vi "Indexer Closed Loop Control.vi"(10 "Indexer backward":bool, 11 "Indexer Forward":bool) -> (3 "Output PWM":dbl)   [LabVIEW 2011]
uses:
  <vilib>/addons/control/pid/NI_PID_pid.lvlib
  <vilib>/addons/control/pid/pid.llb/PID (DBL).vi
panel:
  out "RPM Error Sampled":dbl
  out "Encoder Sample Spped":dbl
  in  "D":dbl
  in  "I":dbl
  in  "P":dbl
  out "RPM Error":dbl
  out "Encoder Set Speed":dbl
  out "Actual Encoder Speed":dbl
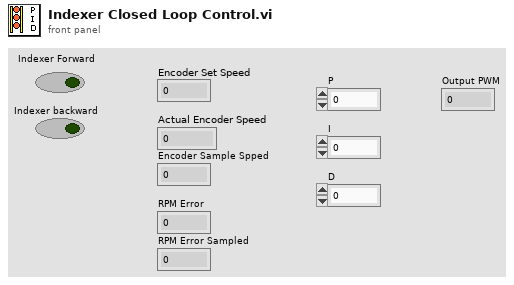
[diagram p1: front panel]
types:
  T1 = typedef "WPI_EncoderDevRef.ctl" = cluster{"DevStatus":errorcluster, "EncoderIndex":T2, "CounterIndex":T3, "DistancePerCount":dbl, "Decoding Type":T4}
  T2 = typedef "FPGA_EncoderIdx.ctl" = enum8{"Enc 0", "Enc 1", "Enc 2", "Enc 3", "Invalid"}
  T3 = typedef "FPGA_CounterCtrSystemIndex.ctl" = enum8{"Ctr 0", "Ctr 1", "Ctr 2", "Ctr 3", "Ctr 4", "Ctr 5", "Ctr 6", "Ctr 7", "Invalid"}
  T4 = typedef "WPI_EncoderType.ctl" = enum16{"1x", "2x", "4x"}
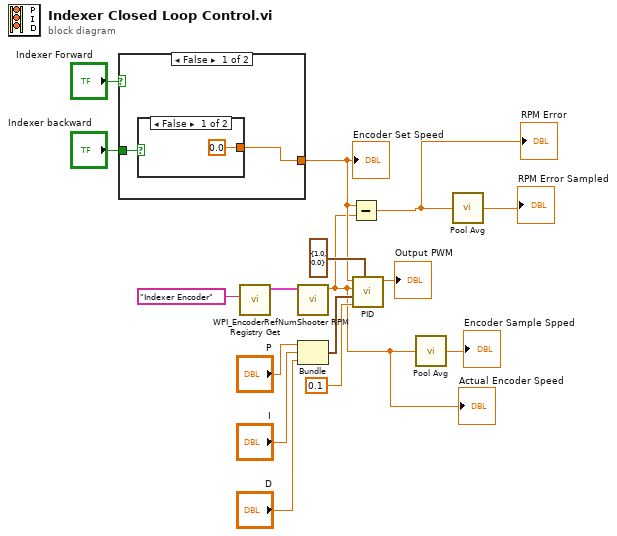
[diagram p0: block diagram]
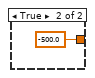
[diagram p2: hidden frame]
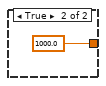
[diagram p3: hidden frame]
diagram:
  n1 = case shown="False" "Indexer Forward" {
    tunnel: [w17 1000.0] -> w11
    tunnel: "Indexer backward" -> [w18 _]
    frame False {
      n2 = case shown="False" w18 {
        tunnel: [0.0 -500.0] -> w17
        frame False {
        }
        frame True {
        }
      }
    }
    frame True {
    }
  }
  "Encoder Set Speed" <- w11
  n3 = call <vilib>:"WPI_EncoderRefNum Registry Get.vi"("refnum name"="Indexer Encoder") -> ("EncoderDevRef"=w6:T1)  [unwired: 9 in, 1 out]
  n4 = call "Shooter RPM.vi"(11:w6) -> ("RPM Output"=w1:dbl)  [unwired: 10 in]
  "Actual Encoder Speed" <- w1
  n5 = Bundle("P"="P", "I"="I", "D"="D") -> (w10:cluster{"P":dbl, "I":dbl, "D":dbl})  [unwired: 1 in]
  n6 = Subtract(x=w11, y=w1) -> (x-y=w3:dbl)
  "RPM Error" <- w3
  n7 = call-poly <vilib>:"PID.vi"("output range"=cluster{"output high":dbl, "output low":dbl} {"output high"=1.0, "output low"=0.0}, "dt (s)"=0.1, "PID gains"=w10, "process variable"=w1, "setpoint"=w11) -> ("output"=→"Output PWM":dbl)  [unwired: 5 in, 1 out]
  n8 = call "Pool Avg.vi"("Input"=w1) -> ("Output Avg"=→"Encoder Sample Spped":dbl)
  n9 = call "Pool Avg.vi"("Input"=w3) -> ("Output Avg"=→"RPM Error Sampled":dbl)
